vi "Evaluate moving condition.vi"(5 "Motor params":T1={"Dirección"=enum."Avance", "Tipo"=enum."Simple", "Velocidad (RPM)"=5.0, "Cantidad de pasos"=1, "Avance (mm)"=0.0, "Pasos por rev"=200.0, "Paso del tonillo"=0.0}, 8 "error in":errorcluster, 9 "Home?":bool, 10 "DAQ ID mod":i32, 11 "current position":dbl) -> (0 "error out":errorcluster, 2 "End-stop?":bool, 3 "Move?":bool)   [LabVIEW 2020, in "GUI.lvlib"]
uses:
  GUI.lvlib
  Support/Motor parameters.ctl
  NI DAQ/NI DAQ.lvlib
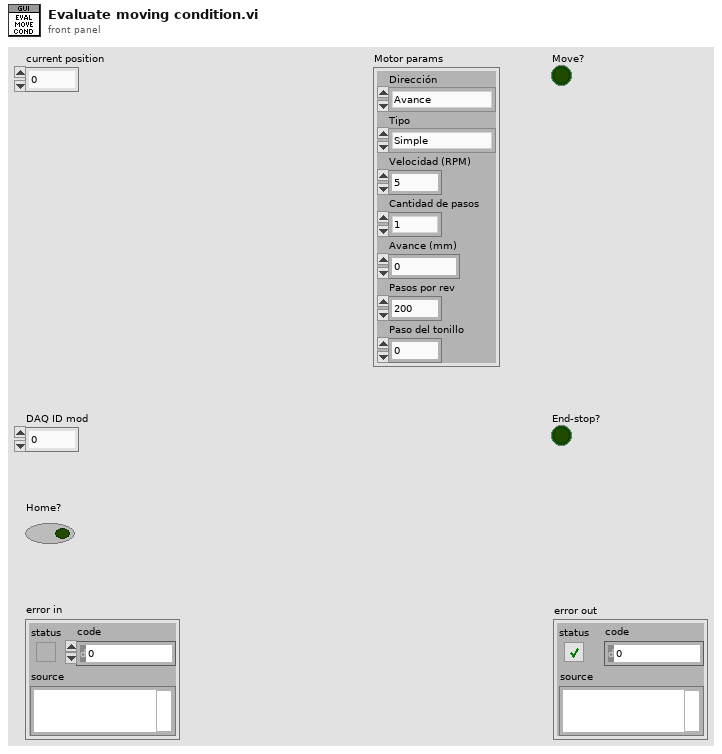
[diagram p1: front panel]
types:
  T1 = typedef "GUI.lvlib/Motor parameters.ctl" = cluster{"Dirección":enum16{"Avance", "Retroceso"}, "Tipo":enum16{"Simple", "Medio paso"}, "Velocidad (RPM)":dbl, "Cantidad de pasos":i32, "Avance (mm)":dbl, "Pasos por rev":dbl, "Paso del tonillo":dbl}
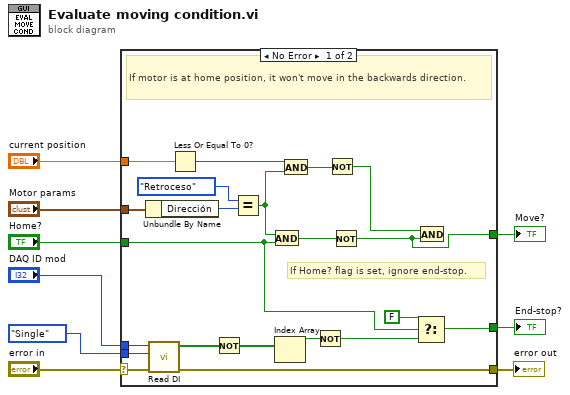
[diagram p0: block diagram]
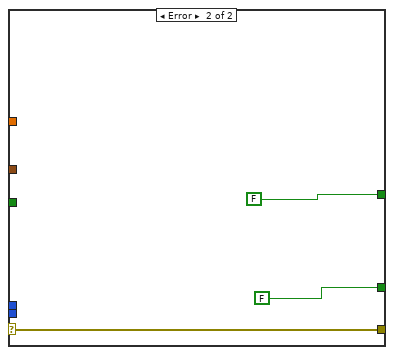
[diagram p2: hidden frame]
diagram:
  n1 = case shown="No Error" "error in" {
    selector: "error in" -> [w26 w33]
    tunnel: "DAQ ID mod" -> [w29 _]
    tunnel: enum16{"Single", "Multiple"}."Single" ("Samples") -> [w28 _]
    tunnel: [w27 w33] -> w8
    tunnel: "Home?" -> [w17 _]
    tunnel: [w10 FALSE] -> w6
    tunnel: "Motor params" -> [w25 _]
    tunnel: [w18 FALSE] -> w2
    tunnel: "current position" -> [w16 _]
    frame No Error {
      # "If Home? flag is set, ignore end-stop."
      # "If motor is at home position, it won't move in the backwards direction."
      n2 = Unbundle By Name(w25) -> ("Dirección"=w24:enum16{"Avance", "Retroceso"})
      n3 = call "Read DI.vi"("error in"=w26, "Samples"=w28, "Module ID"=w29) -> ("error out"=w27:errorcluster, "Data"=w30:bool[])  [unwired: 6 in, 1 out]
      n4 = Less Or Equal To 0?(x=w16) -> (x <= 0?=w15:bool)
      n5 = Not(x=w30) -> (.not. x?=w11:bool[])
      n6 = Equal?(x=enum16{"Avance", "Retroceso"}."Retroceso", y=w24) -> (x = y?=w14:bool)
      n7 = And(x=w14, y=w17) -> (x .and. y?=w21:bool)
      n8 = Index Array(array=w11) -> (element=w22:bool)  [unwired: 1 in]
      n9 = And(x=w15, y=w14) -> (x .and. y?=w13:bool)
      n10 = Not(x=w22) -> (.not. x?=w19:bool)
      n11 = Not(x=w13) -> (.not. x?=w12:bool)
      n12 = Not(x=w21) -> (.not. x?=w10:bool)
      n13 = Select(t=FALSE, s=w17, f=w19) -> (s? t:f=w18:bool)
      n14 = And(x=w12, y=w10) -> ()  [unwired: 1 out]
    }
    frame Error {
    }
  }
  "error out" <- w8
  "Move?" <- w6
  "End-stop?" <- w2
